vi "remove.invalid.chars.vi"(1 "string in":string) -> (0 "string out":string)   [LabVIEW 2024]
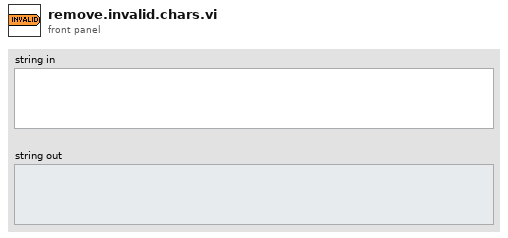
[diagram p1: front panel]
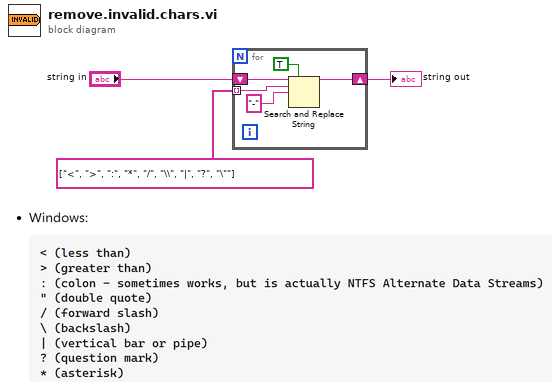
[diagram p0: block diagram]
diagram:
  n1 = for {
    shift-right: [w7] -> w2
    shift-left: "string in" -> [w8]
    tunnel: string[] ["<", ">", ":", "*", "/", "\\", "|", "?", "\""] -> [w6] mode=indexing
    n2 = Search and Replace String(replace all?=TRUE ("replace all? (F)"), input string=w8, search string=w6, replace string="-" ("replace string (\"\")")) -> (result string=w7:string)  [unwired: 4 in, 3 out]
  }
  "string out" <- w2
